vi "set Data Element.vi"(0 "LVx - Template Command in":refnum<class "LVx - Template Command.lvclass">, 5 "Test String":T1, 11 "error in (no error)":errorcluster) -> (4 "LVx - Template Command out":refnum<class "LVx - Template Command.lvclass">, 15 "error out":errorcluster)   [LabVIEW 2011, in "LVx.lvlib" / "LVx - Template Command.lvclass"]
uses:
  LVx - Template Command.lvclass
  Command Data Element.ctl
  LVx - Template Command.lvclass/LVx - Template Command.ctl
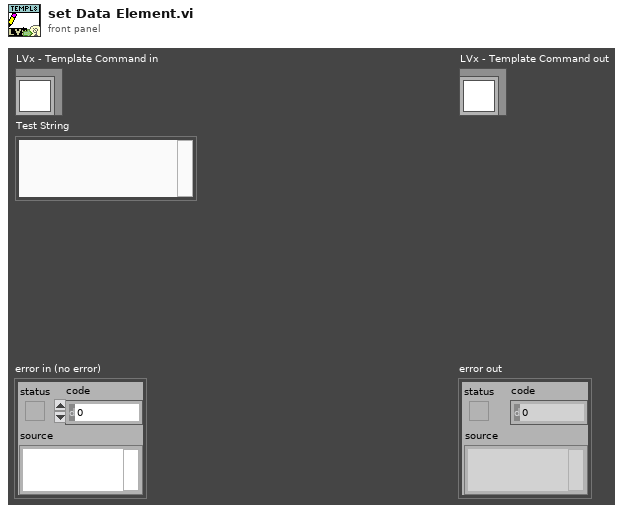
[diagram p1: front panel]
types:
  T1 = typedef "LVx.lvlib/LVx - Template Command.lvclass/Command Data Element.ctl" = string
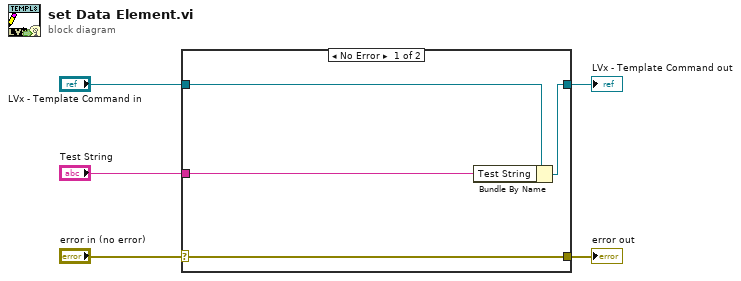
[diagram p0: block diagram]
diagram:
  n1 = case shown="No Error" "error in (no error)" {
    selector: "error in (no error)" -> [w9 w10]
    tunnel: [w9 w10] -> w4
    tunnel: [w7 w11] -> w2
    tunnel: "LVx - Template Command in" -> [w8 w11]
    tunnel: "Test String" -> [w6 _]
    frame No Error {
      n2 = Bundle By Name(cluster=w8, "Test String"=w6) -> (w7:refnum<class "LVx - Template Command.lvclass">)
    }
    frame Error {
    }
  }
  "error out" <- w4
  "LVx - Template Command out" <- w2
